vi "Init.vi"(8 "error in (no error)":errorcluster, 10 "ID":string, 11 "Actuator in":refnum<class "Actuator.lvclass">) -> (0 "error out":errorcluster, 3 "Actuator out":refnum<class "Actuator.lvclass">)   [LabVIEW 2021, in "Actuator.lvclass"]
uses:
  Actuator.lvclass
  Actuator.lvclass/Actuator.ctl
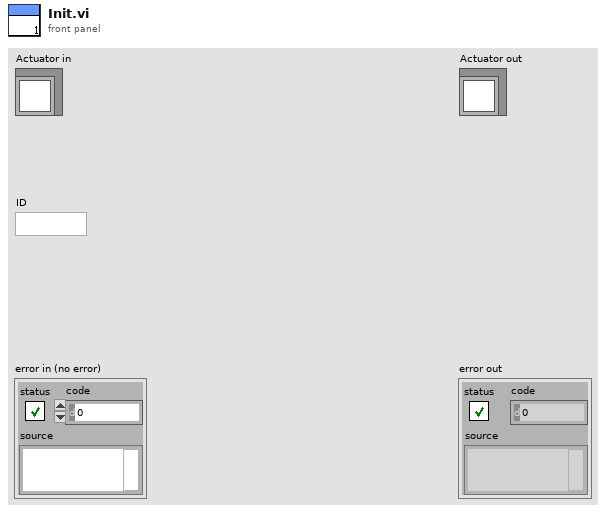
[diagram p1: front panel]
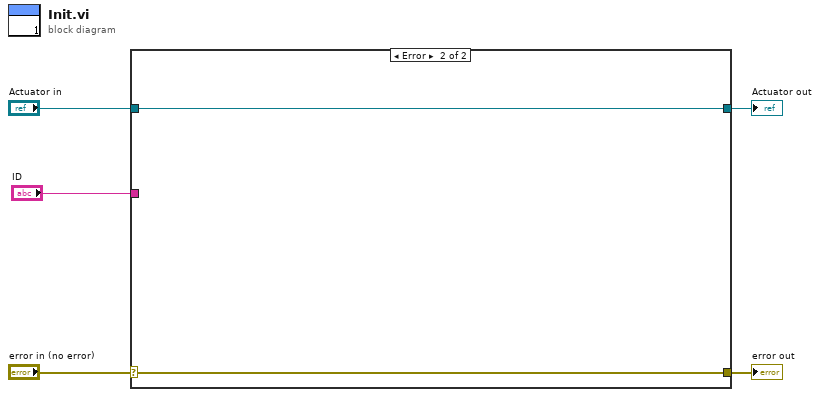
[diagram p0: block diagram]
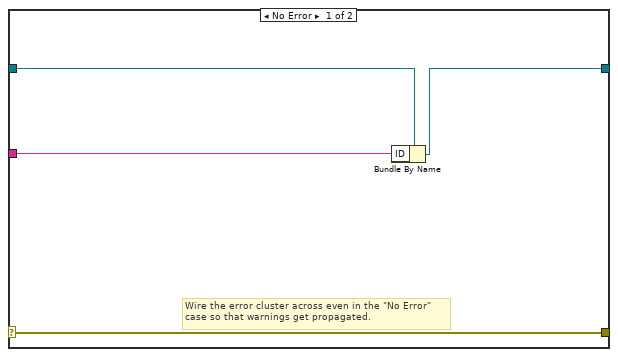
[diagram p2: hidden frame]
diagram:
  n1 = case shown="Error" "error in (no error)" {
    selector: "error in (no error)" -> [w9 w11]
    tunnel: [w9 w11] -> w4
    tunnel: [w8 w10] -> w2
    tunnel: "Actuator in" -> [w7 w10]
    tunnel: "ID" -> [w6 _]
    frame No Error {
      # "Wire the error cluster across even in the \"No Error\"\ncase so that warnings get propagated."
      n2 = Bundle By Name(cluster=w7, "ID"=w6) -> (w8:refnum<class "Actuator.lvclass">)
    }
    frame Error {
    }
  }
  "error out" <- w4
  "Actuator out" <- w2
